vi "Search Direction Array.vi"(10 "Target Items":T1[](array[typedef]), 11 "Search Array":T1[](array[typedef])) -> (2 "Found Direction":T1, 3 "Found":bool)   [LabVIEW 2017, in "AntFarm_MB.lvclass"]
uses:
  AntFarm_MB.lvclass
  Type Defs/Direction Enum.ctl
  Type Defs/SB Type Defs.lvlib
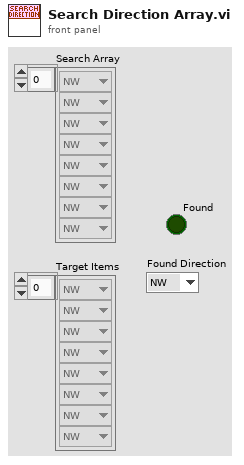
[diagram p1: front panel]
types:
  T1 = typedef "SB Type Defs.lvlib/Direction Enum.ctl" = enum16{"NW", "N", "NE", "E", "SE", "S", "SW", "W"}
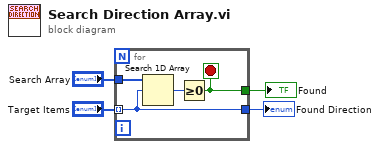
[diagram p0: block diagram]
diagram:
  n1 = for {
    tunnel: "Search Array" -> [w8]
    tunnel: "Target Items" -> [w6] mode=indexing
    tunnel: [w6] -> w3
    tunnel: [w5] -> w4
    stop <- w5 stop-if-true
    n2 = Search 1D Array(1D array=w8, element=w6) -> (index of element=w7:i32)  [unwired: 1 in]
    n3 = Greater Or Equal To 0?(x=w7) -> (x >= 0?=w5:bool)
  }
  "Found" <- w4
  "Found Direction" <- w3
